vi "DrawLine.vi"(8 "error in":errorcluster, 10 "Line":T1, 11 "FPGA VI Reference In":T3) -> (0 "error out":errorcluster, 3 "FPGA VI Reference Out":T3)   [LabVIEW 2019]
uses:
  TypeDefs/FPGA Reference.ctl
  TypeDefs/Line.ctl
  TypeDefs/Pixel.ctl
panel:
  out "Y":i16[](array[numeric])
  out "X":i32[](array[numeric])
  out "x-y":i16
  in  "Color":u16=65535 format="%.0x"
  out "Array":u16[][](array[numeric]) format="%.0x"
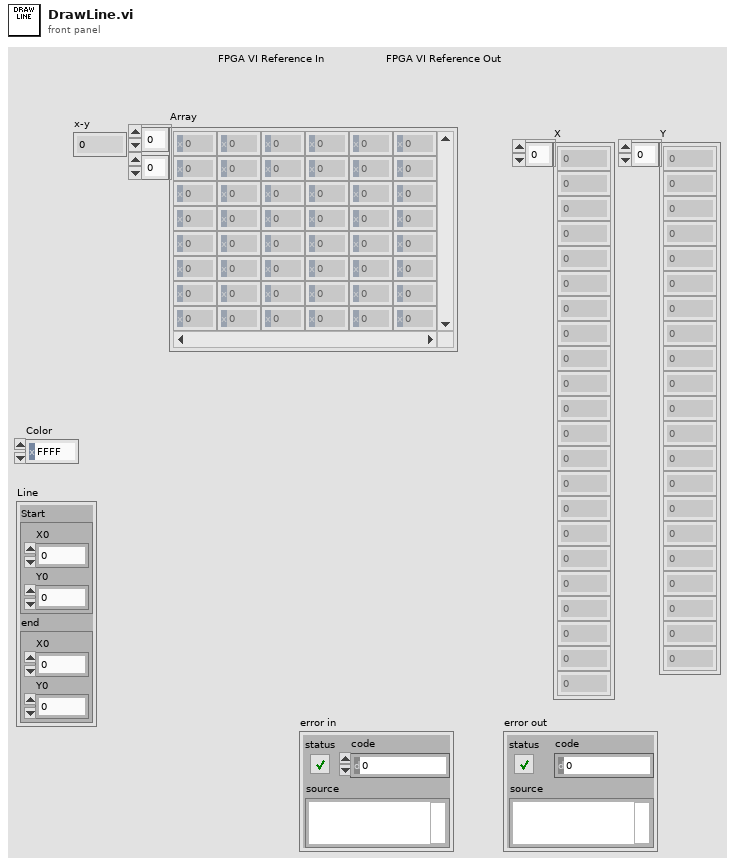
[diagram p1: front panel]
types:
  T1 = typedef "Line.ctl" = cluster{"Start":T2, "end":T2}
  T2 = typedef "Pixel.ctl" = cluster{"X0":i16, "Y0":i16}
  T3 = typedef "FPGA Reference.ctl" = refnum<k20>
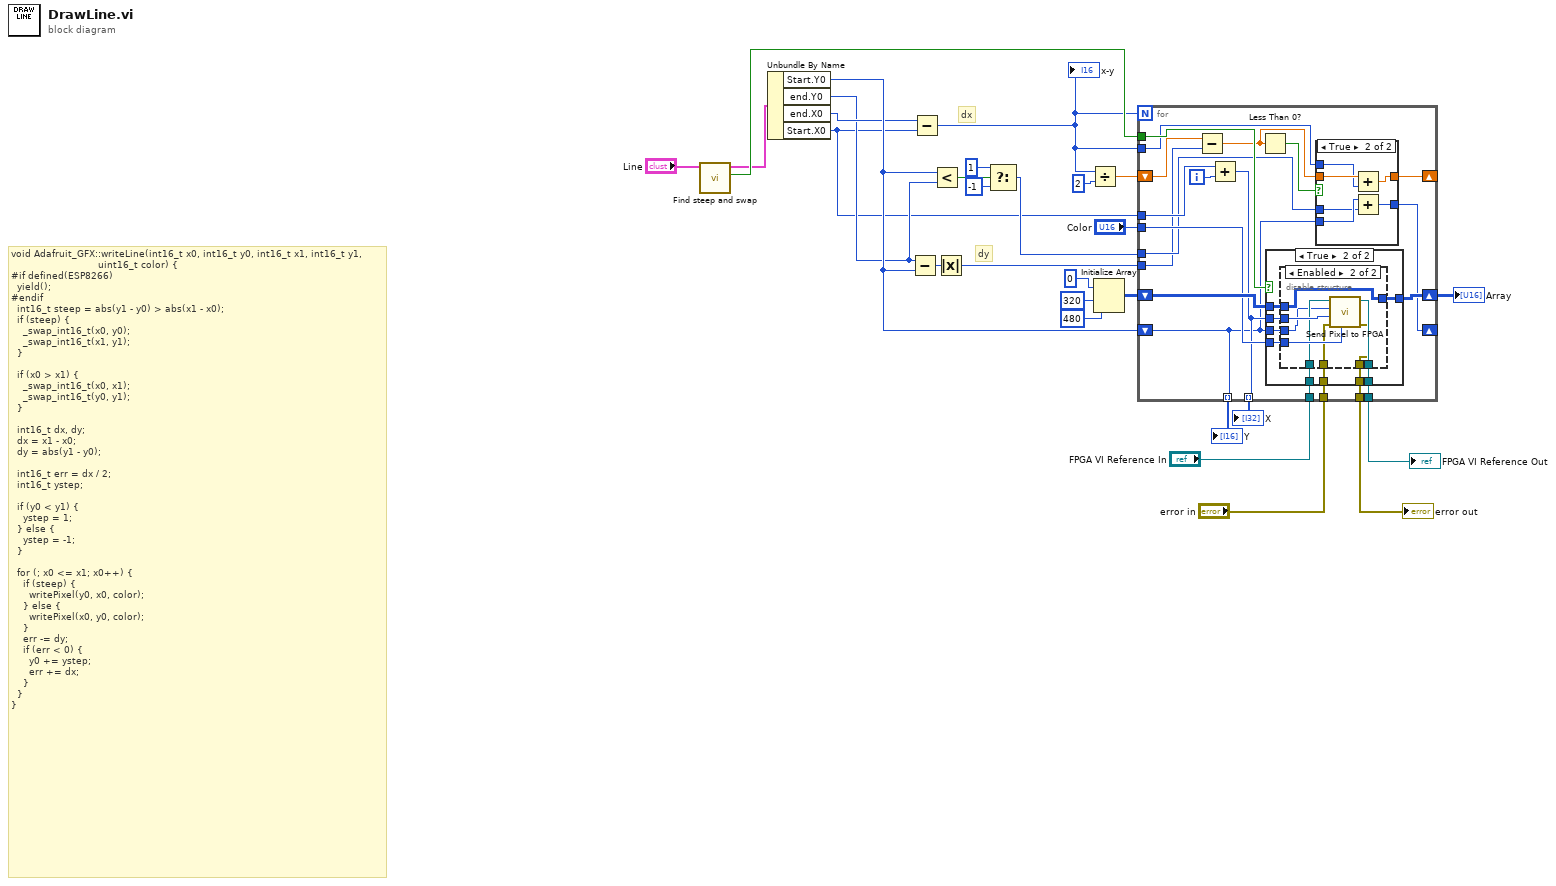
[diagram p0: block diagram]
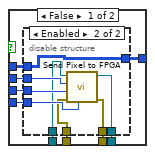
[diagram p3: hidden frame]
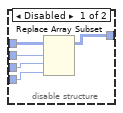
[diagram p4: hidden frame]
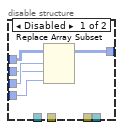
[diagram p5: hidden frame]
diagram:
  # "dy"
  # "dx"
  # "void Adafruit_GFX::writeLine(int16_t x0, int16_t y0, int16_t x1, int16_t y1,\n                             uint16_t color) {\n#if defined(ESP8266)\n  yield();\n#endif\n  int16_t steep = abs(y1 - y0) > abs(x1 - x0);\n  if (steep) {\n    _swap_int16_t(x0, y0);\n    _swap_int16_t(x1, y1);\n  }\n\n  if (x0 > x1) {\n    _swap_int16_t(x0, x1);\n    _swap_int16_t(y0, y1);\n  }\n\n  int16_t dx, dy;\n  dx = x1 - x0;\n  dy = abs(y1 - y0);\n\n  int16_t err = dx / 2;\n  int16_t ystep;\n\n  if (y0 < y1) {\n    ystep = 1;\n  } else {\n    ystep = -1;\n  }\n\n  for (; x0 <= x1; x0++) {\n    if (steep) {\n      writePixel(y0, x0, color);\n    } else {\n      writePixel(x0, y0, color);\n    }\n    err -= dy;\n    if (err < 0) {\n      y0 += ystep;\n      err += dx;\n    }\n  }\n}"
  n1 = call "Find steep and swap.vi"("Line"="Line") -> ("steep"=w23:bool, "Line Out"=w7:T1)  [unwired: 9 in]
  n2 = Unbundle By Name(w7) -> ("Start.Y0"=w6:i16, "end.Y0"=w4:i16, "end.X0"=w5:i16, "Start.X0"=w3:i16)
  n3 = Subtract(x=w4, y=w6) -> (x-y=w17:i16)
  n4 = Subtract(x=w5, y=w3) -> (x-y=w16:i16)
  "x-y" <- w16
  n5 = Less?(x=w6, y=w4) -> (x < y?=w26:bool)
  n6 = Absolute Value(x=w17) -> (abs(x)=w15:i16)
  n7 = Select(t=i16 1, s=w26, f=i16 -1 ("t")) -> (s? t:f=w19:i16)
  n8 = Divide(x=w16, y=i16 2) -> (x/y=w18:dbl)
  n9 = Initialize Array(u16 0, 320 ("dimension size"), 480 ("dimension size")) -> (w22:u16[][])
  n10 = for {
    N: w16 -> [_]
    tunnel: w3 -> [w48]
    tunnel: w23 -> [w43]
    shift-right: [w45] -> w20
    shift-left: w22 -> [w46]
    tunnel: "Color" -> [w44]
    tunnel: w15 -> [w40]
    shift-right: [w38] -> _
    shift-left: w6 -> [w29]
    tunnel: w19 -> [w42]
    shift-right: [w35] -> _
    shift-left: w18 -> [w41]
    tunnel: w16 -> [w36]
    tunnel: "FPGA VI Reference In" -> [w34]
    tunnel: [w33] -> w13
    tunnel: "error in" -> [w32]
    tunnel: [w31] -> w11
    tunnel: [w30] -> w2 mode=indexing
    tunnel: [w29] -> w1 mode=indexing
    i -> [w47]
    n11 = Subtract(x=w41, y=w40) -> (x-y=w37:dbl)
    n12 = Add(x=w48, y=w47) -> (x+y=w30:i32)
    n13 = Less Than 0?(x=w37) -> (x < 0?=w39:bool)
    n14 = case shown="True" w43 {
      tunnel: w46 -> [w65 w87]
      tunnel: [w64 w86] -> w45
      tunnel: w30 -> [w63 w83]
      tunnel: w29 -> [w62 w84]
      tunnel: w44 -> [w61 w85]
      tunnel: w34 -> [w60 w82]
      tunnel: [w59 w81] -> w33
      tunnel: w32 -> [w57 w80]
      tunnel: [w58 w79] -> w31
      frame False {
        n15 = disable-structure shown="Enabled" {
          disable-tunnel: w65 -> [w70 w71]
          disable-tunnel: [w69 w71] -> w64
          disable-tunnel: w63 -> [w68 w78]
          disable-tunnel: w62 -> [w67 w77]
          disable-tunnel: w61 -> [w66 w76]
          disable-tunnel: w60 -> [_ w75]
          disable-tunnel: [_ w74] -> w59
          disable-tunnel: [_ w73] -> w58
          disable-tunnel: w57 -> [_ w72]
          frame Disabled {
            n16 = Replace Array Subset(array=w70, new element=w66, index (row)=w68, index (col)=w67) -> (w69:u16[][])
          }
          frame Enabled {
            n17 = call "Send Pixel to FPGA.vi"("Color"=w76, "error in"=w72, "Y"=w77, "X"=w78, "FPGA VI Reference Out"=w75) -> ("error out"=w73:errorcluster, "FPGA VI Reference Out 2"=w74:T3)  [unwired: 5 in]
          }
        }
      }
      frame True {
        n18 = disable-structure shown="Enabled" {
          disable-tunnel: w87 -> [w92 w94]
          disable-tunnel: [w91 w94] -> w86
          disable-tunnel: w85 -> [w90 w99]
          disable-tunnel: w84 -> [w89 w93]
          disable-tunnel: w83 -> [w88 w100]
          disable-tunnel: w82 -> [_ w98]
          disable-tunnel: [_ w97] -> w81
          disable-tunnel: w80 -> [_ w96]
          disable-tunnel: [_ w95] -> w79
          frame Disabled {
            n19 = Replace Array Subset(array=w92, new element=w90, index (row)=w89, index (col)=w88) -> (w91:u16[][])
          }
          frame Enabled {
            n20 = call "Send Pixel to FPGA.vi"("Color"=w99, "error in"=w96, "Y"=w100, "X"=w93, "FPGA VI Reference Out"=w98) -> ("error out"=w95:errorcluster, "FPGA VI Reference Out 2"=w97:T3)  [unwired: 5 in]
          }
        }
      }
    }
    n21 = case shown="True" w39 {
      tunnel: w29 -> [w49 w56]
      tunnel: w42 -> [_ w55]
      tunnel: [w49 w54] -> w38
      tunnel: w37 -> [w50 w53]
      tunnel: w36 -> [_ w52]
      tunnel: [w50 w51] -> w35
      frame False {
      }
      frame True {
        n22 = Add(x=w53, y=w52) -> (x+y=w51:dbl)
        n23 = Add(x=w56, y=w55) -> (x+y=w54:i16)
      }
    }
  }
  "Array" <- w20
  "FPGA VI Reference Out" <- w13
  "error out" <- w11
  "X" <- w2
  "Y" <- w1
